vi "FTP.Flush.vi"(8 "error in (no error)":errorcluster, 10 "host":string) -> (0 "error out":errorcluster, 3 "FTP Session out":T1)   [LabVIEW 2016]
uses:
  <vilib>/FTP/ftp0.llb/FTP Session.ctl
  <vilib>/FTP/NI_FTP.lvlib
panel:
  out "Files":string[](array[string])
  in  "remote port (21)":u16=21
  in  "password":string="admin"
  in  "user":string="admin"
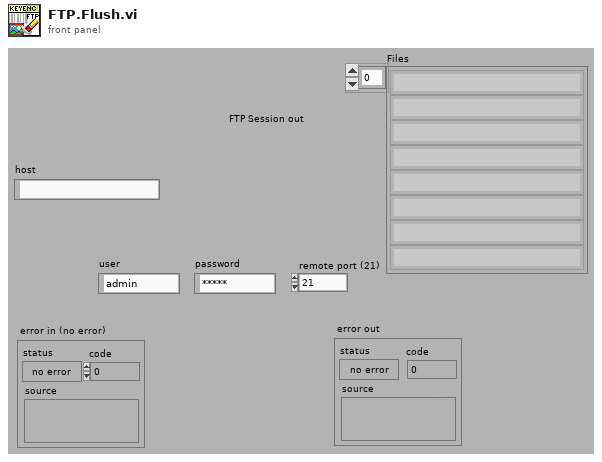
[diagram p1: front panel]
types:
  T1 = typedef "NI_FTP.lvlib/FTP Session.ctl" = refnum<k5>
  T2 = typedef "NI_FTP.lvlib/FTP File Info.ctl" = cluster{"type":enum16{"unknown", "file", "dir", "link"}, "permissions":string, "owner":string, "group":string, "size":i32, "date":string, "name":string, "link name":string}
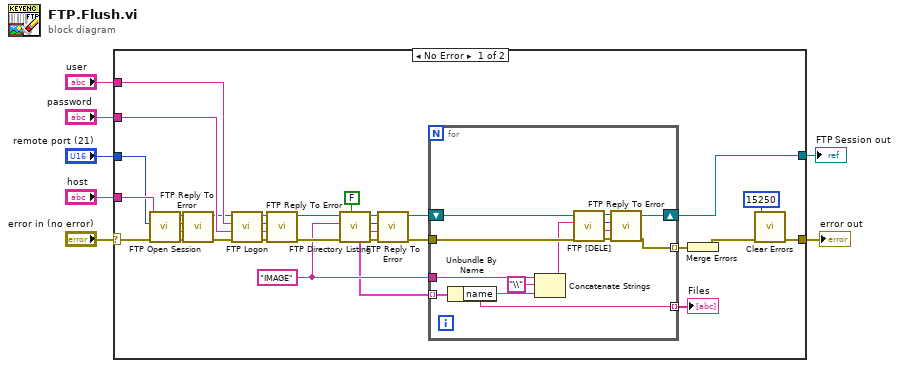
[diagram p0: block diagram]
diagram:
  n1 = case shown="No Error" "error in (no error)" {
    selector: "error in (no error)" -> [w18 w53]
    tunnel: "host" -> [w39 _]
    tunnel: "user" -> [w38 _]
    tunnel: "password" -> [w37 _]
    tunnel: "remote port (21)" -> [w26 _]
    tunnel: [w9 w53] -> w3
    tunnel: [w11 _] -> w1
    frame No Error {
      w16 = "IMAGE" ("directory path")
      n2 = call <vilib>:"FTP Open Session.vi"("error in (no error)"=w18, "remote port (21)"=w26, "address"=w39) -> ("error out"=w36:errorcluster, "reply string"=w33:string, "reply code"=w34:i32, "ftp session"=w35:T1)  [unwired: 5 in]
      n3 = call <vilib>:"FTP Reply To Error.vi"("error in (no error)"=w36, "reply string in"=w33, "reply code in"=w34, "ftp session"=w35) -> ("error out"=w31:errorcluster, "ftp session out"=w32:T1)  [unwired: 2 out]
      n4 = call <vilib>:"FTP Logon.vi"("error in (no error)"=w31, "password"=w37, "user"=w38, "ftp session"=w32) -> ("error out"=w30:errorcluster, "reply string"=w27:string, "reply code"=w28:i32, "ftp session out"=w29:T1)  [unwired: 4 in]
      n5 = call <vilib>:"FTP Reply To Error.vi"("error in (no error)"=w30, "reply string in"=w27, "reply code in"=w28, "ftp session"=w29) -> ("error out"=w19:errorcluster, "ftp session out"=w20:T1)  [unwired: 2 out]
      n6 = call <vilib>:"FTP Directory Listing.vi"("active (T)"=FALSE, "error in (no error)"=w19, "directory path"=w16, "ftp session"=w20) -> ("error out"=w24:errorcluster, "reply string"=w22:string, "reply code"=w23:i32, "ftp session out"=w25:T1, "dir list"=w15:T2[])  [unwired: 3 in]
      n7 = call <vilib>:"FTP Reply To Error.vi"("error in (no error)"=w24, "reply string in"=w22, "reply code in"=w23, "ftp session"=w25) -> ("error out"=w14:errorcluster, "ftp session out"=w13:T1)  [unwired: 2 out]
      n8 = for {
        tunnel: w14 -> [w52]
        tunnel: w15 -> [w46] mode=indexing
        tunnel: w16 -> [w45]
        tunnel: [w43] -> w17 mode=indexing
        shift-right: [w42] -> w11
        shift-left: w13 -> [w51]
        tunnel: [w40] -> w12 mode=indexing
        n9 = Unbundle By Name(w46) -> ("name"=w40:string)
        n10 = Concatenate Strings(w45, "\\" ("string"), w40) -> (w41:string)
        n11 = call <vilib>:"FTP [DELE].vi"("error in (no error)"=w52, "file path"=w41, "ftp session"=w51) -> ("error out"=w50:errorcluster, "reply string"=w47:string, "reply code"=w48:i32, "ftp session out"=w49:T1)  [unwired: 5 in]
        n12 = call <vilib>:"FTP Reply To Error.vi"("error in (no error)"=w50, "reply string in"=w47, "reply code in"=w48, "ftp session"=w49) -> ("error out"=w43:errorcluster, "ftp session out"=w42:T1)  [unwired: 2 out]
      }
      "Files" <- w12
      n13 = Merge Errors(w17) -> (w10:errorcluster)
      n14 = call <vilib>:"Clear Errors.vi"("error in (no error)"=w10, "specific error code to clear (0: all)"=15250) -> ("error out"=w9:errorcluster)  [unwired: 4 in, 1 out]
    }
    frame Error {
    }
  }
  "error out" <- w3
  "FTP Session out" <- w1
